vi "6221+5650.vi"() -> ()   [LabVIEW 2019]
uses:
  <vilib>/Utility/file.llb/Write Delimited Spreadsheet (string).vi
  SubVI/SubVI.lvlib
panel:
  in  "file path (use dialog)":path
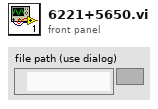
[diagram p1: front panel]
types:
  T1 = enum16{"open", "replace", "create", "open or create", "replace or create", "replace or create with confirmation"}
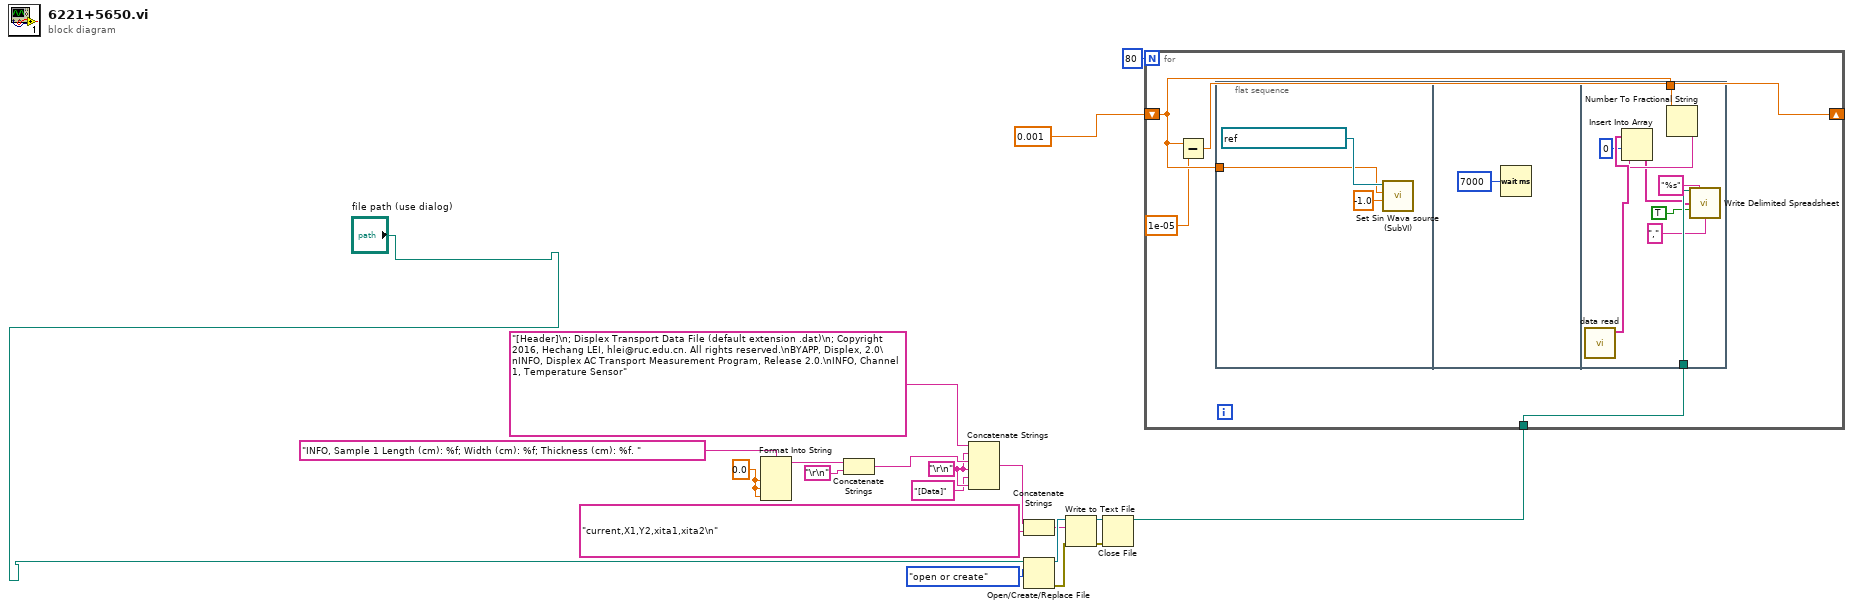
[diagram p0: block diagram]
diagram:
  w9 = 0.0 ("输入 1")
  w12 = "\r\n"
  n1 = Format Into String(format string="INFO, Sample 1 Length (cm): %f; Width (cm): %f; Thickness (cm): %f. " ("string"), w9, w9, w9) -> (resulting string=w16:string)  [unwired: 2 in, 1 out]
  n2 = Concatenate Strings(w16, "\r\n") -> (w17:string)
  n3 = Concatenate Strings("[Header]\n; Displex Transport Data File (default extension .dat)\n; Copyright 2016, Hechang LEI, hlei@ruc.edu.cn. All rights reserved.\nBYAPP, Displex, 2.0\nINFO, Displex AC Transport Measurement Program, Release 2.0.\nINFO, Channel 1, Temperature Sensor" ("string"), w12, w17, w12, "[Data]" ("string"), w12) -> (w18:string)
  n4 = Concatenate Strings(w18, "current,X1,Y2,xita1,xita2\n" ("字符串")) -> (w8:string)
  n5 = Open/Create/Replace File(file path (use dialog)="file path (use dialog)", operation (0:open)=T1."open or create") -> (refnum out=w19:refnum<file>, error out=w5:errorcluster)  [unwired: 4 in, 1 out]
  n6 = Write to Text File(file (use dialog)=w19, text=w8, error in=w5) -> (refnum out=w7:refnum<file>, error out=w6:errorcluster)  [unwired: 1 in, 1 out]
  n7 = Close File(refnum=w7, error in=w6) -> (path=w4:path)  [unwired: 1 out]
  n8 = for {
    N: 80 -> [_]
    tunnel: w4 -> [w24]
    shift-right: [w23] -> _
    shift-left: 0.001 -> [w22]
    n9 = Subtract(x=w22, y=1e-05 ("x")) -> (x-y=w23:dbl)
    n10 = flat-sequence {
      tunnel: w22 -> [w25]
      tunnel: w24 -> [w37]
      tunnel: w22 -> [w31]
      frame #0 {
        n11 = call "Set Sin Wava source (SubVI).vi"("Hz"=-1.0, "A"=w25, "VISA引用句柄输入"=refnum<visa-resource-name> "GPIB0::10::INSTR") -> ()  [unwired: 9 in]
      }
      frame #1 {
        n12 = Wait (ms)(milliseconds to wait=u32 7000) -> ()  [unwired: 1 out]
      }
      frame #2 {
        n13 = call "data read.vi"() -> ("F-format string"=w33:string[])  [unwired: 11 in]
        n14 = Number To Fractional String(number=w31) -> (F-format string=w30:string)  [unwired: 3 in]
        n15 = Insert Into Array(array=w33, index=0, new element=w30) -> (w29:string[])
        n16 = call-poly <vilib>:"Write Delimited Spreadsheet.vi"("file path (dialog if empty)"=w37, "format (%s)"="%s" ("format (%.3f)"), "1D data"=w29, "append to file? (new file:F)"=TRUE, "delimiter (\\t)"="," ("delimiter (\\t)")) -> ()  [unwired: 9 in, 2 out]
      }
    }
  }
